vi "AddBusPark.vi"(8 "error in (no error)":errorcluster, 9 "Number of Samples In":i32, 10 "Data Array In":u8[][](array[numeric]), 11 "RFFE_Data In":T1 {"Toggle (high to low)" items=["0", "1", "Z", "L", "H", "X", "T", "V"]; "X Array" items=["0", "1", "Z", "L", "H", "X", "T", "V"]; "Z Array" items=["0", "1", "Z", "L", "H", "X", "T", "V"]; "L Array" items=["0", "1", "Z", "L", "H", "X", "T", "V"]; "H Array" items=["0", "1", "Z", "L", "H", "X", "T", "V"]; "One Array" items=["0", "1", "Z", "L", "H", "X", "T", "V"]; "Zero Array" items=["0", "1", "Z", "L", "H", "X", "T", "V"]}) -> (0 "error out":errorcluster, 1 "Number of Samples Out":i32, 2 "Data Array Out":u8[][](array[numeric]), 3 "RFFE_Data Out":T1 {"Toggle (high to low)" items=["0", "1", "Z", "L", "H", "X", "T", "V"]; "X Array" items=["0", "1", "Z", "L", "H", "X", "T", "V"]; "Z Array" items=["0", "1", "Z", "L", "H", "X", "T", "V"]; "L Array" items=["0", "1", "Z", "L", "H", "X", "T", "V"]; "H Array" items=["0", "1", "Z", "L", "H", "X", "T", "V"]; "One Array" items=["0", "1", "Z", "L", "H", "X", "T", "V"]; "Zero Array" items=["0", "1", "Z", "L", "H", "X", "T", "V"]})   [LabVIEW 2013]
doc: "Builds MIPI RFFE bus park"
uses:
  Ctrls/RFFE_Data.ctl
  Ctrls/ClockDataChannels.ctl
  Ctrls/BitStates.ctl
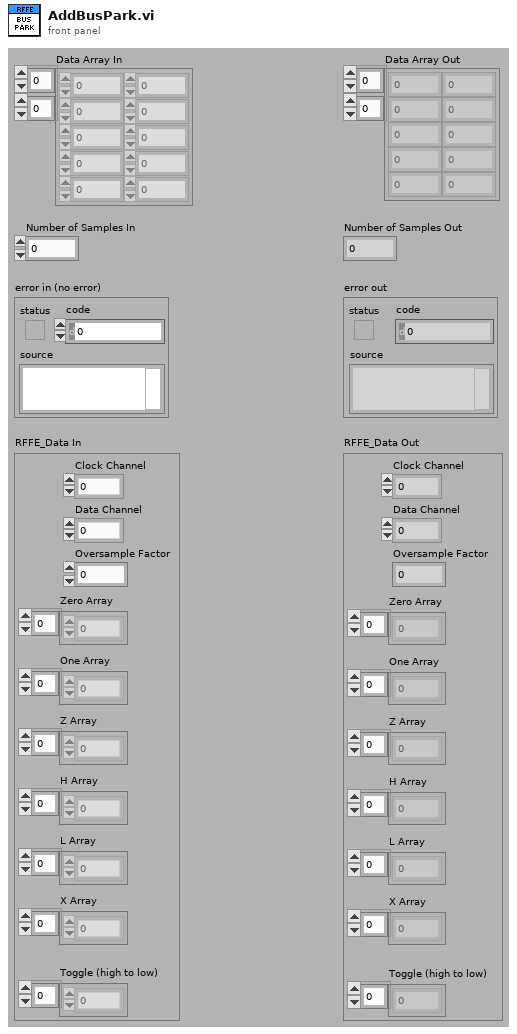
[diagram p1: front panel]
types:
  T1 = typedef "RFFE_Data.ctl" = cluster{"Clock Channel":T2, "Data Channel":T2, "Oversample Factor":u8, "Zero Array":u8[], "One Array":u8[], "Z Array ":u8[], "H Array":u8[], "L Array":u8[], "X Array":u8[], "Toggle (high to low)":u8[]}
  T2 = typedef "ClockDataChannels.ctl" = enum16{"0", "1"}
  T3 = typedef "BitStates.ctl" = enum16{"0", "1", "Z", "L", "H", "X", "Toggle"}
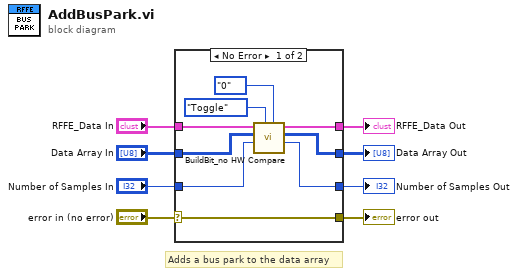
[diagram p0: block diagram]
diagram:
  # "Adds a bus park to the data array"
  n1 = case shown="No Error" "error in (no error)" {
    selector: "error in (no error)" -> [w17 w18]
    tunnel: [w17 w18] -> w7
    tunnel: [w11 w21] -> w6
    tunnel: "RFFE_Data In" -> [w12 w21]
    tunnel: [w10 w20] -> w5
    tunnel: "Data Array In" -> [w16 w20]
    tunnel: "Number of Samples In" -> [w15 w19]
    tunnel: [w9 w19] -> w1
    frame No Error {
      n2 = call "BuildBit_no HW Compare.vi"("Data Value"=BitStates."0", "Clock Value"=BitStates."Toggle", "Number of Samples In"=w15, "Data Array In"=w16, "RFFE_Data In"=w12) -> ("Number of Samples Out"=w9:i32, "Data Array Out"=w10:u8[][], "RFFE_Data Out"=w11:T1)  [unwired: 4 in]
    }
    frame Error {
    }
  }
  "error out" <- w7
  "RFFE_Data Out" <- w6
  "Data Array Out" <- w5
  "Number of Samples Out" <- w1
